vi "SaveFramWriteTDMS.vi"(0 "object in":refnum<class "Hamamatsu.lvclass">, 1 "Image":T1, 2 "base path":path, 3 "FrameIdx":i32, 4 "tdms file":refnum<k34>, 5 "error in (no error)":errorcluster, 7 "group name":string) -> (14 "object out":refnum<class "Hamamatsu.lvclass">, 19 "error out":errorcluster)   [LabVIEW 2023, in "Hamamatsu.lvclass"]
uses:
  Hamamatsu.lvclass
  <vilib>/vision/Image Controls.llb/IMAQ Image.ctl
  Hamamatsu.lvclass/Hamamatsu.ctl
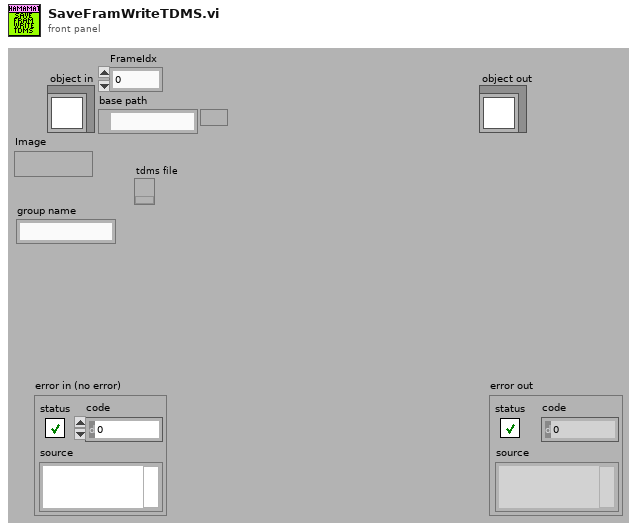
[diagram p1: front panel]
types:
  T1 = typedef "IMAQ Image.ctl" = refnum<image>
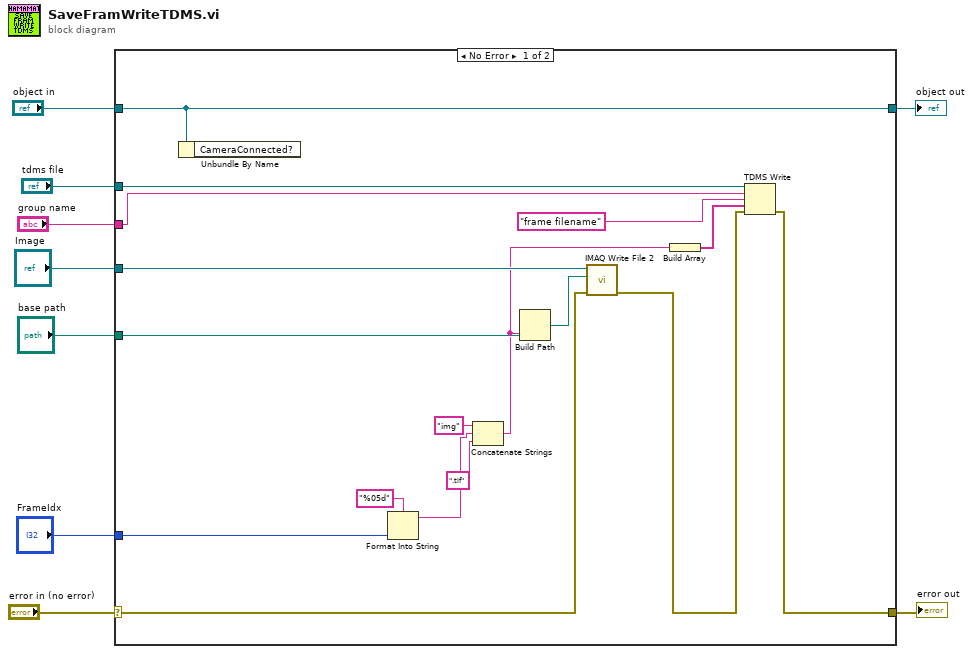
[diagram p0: block diagram]
diagram:
  n1 = case shown="No Error" "error in (no error)" {
    selector: "error in (no error)" -> [w17 w28]
    tunnel: [w14 w28] -> w8
    tunnel: [w26 w27] -> w6
    tunnel: "object in" -> [w26 w27]
    tunnel: "Image" -> [w25 _]
    tunnel: "FrameIdx" -> [w23 _]
    tunnel: "base path" -> [w19 _]
    tunnel: "tdms file" -> [w16 _]
    tunnel: "group name" -> [w13 _]
    frame No Error {
      n2 = Unbundle By Name(w26) -> ()  [unwired: 1 out]
      n3 = Format Into String(format string="%05d", w23) -> (resulting string=w21:string)  [unwired: 2 in, 1 out]
      n4 = Concatenate Strings("img" ("string"), w21, ".tif" ("string")) -> (w10:string)
      n5 = Build Path(base path=w19, name or relative path=w10) -> (appended path=w18:path)
      n6 = call-poly "IMAQ Write File 2"("error in (no error)"=w17, "File Path"=w18, "Image"=w25) -> ("error out"=w15:errorcluster)  [unwired: 7 in, 1 out]
      n7 = Build Array(w10) -> (w11:string[])
      n8 = TDMS Write(0:w16, 5:w13, 7:"frame filename", 9:w11, 11:w15) -> (15:w14:errorcluster)  [unwired: 1 in, 3 out]
    }
    frame Error {
    }
  }
  "error out" <- w8
  "object out" <- w6
